vi "String_parsingV3.vi"(4 "input string":string) -> (0 "V3":i32[](array[numeric]), 1 "V2":i32[](array[numeric]), 2 "V1":i32[](array[numeric]))   [LabVIEW 2014]
panel:
  out "size(s)":i32
  out "input test":u8[](array[numeric])
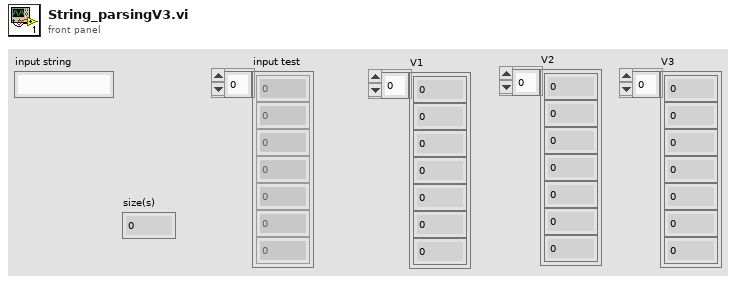
[diagram p1: front panel]
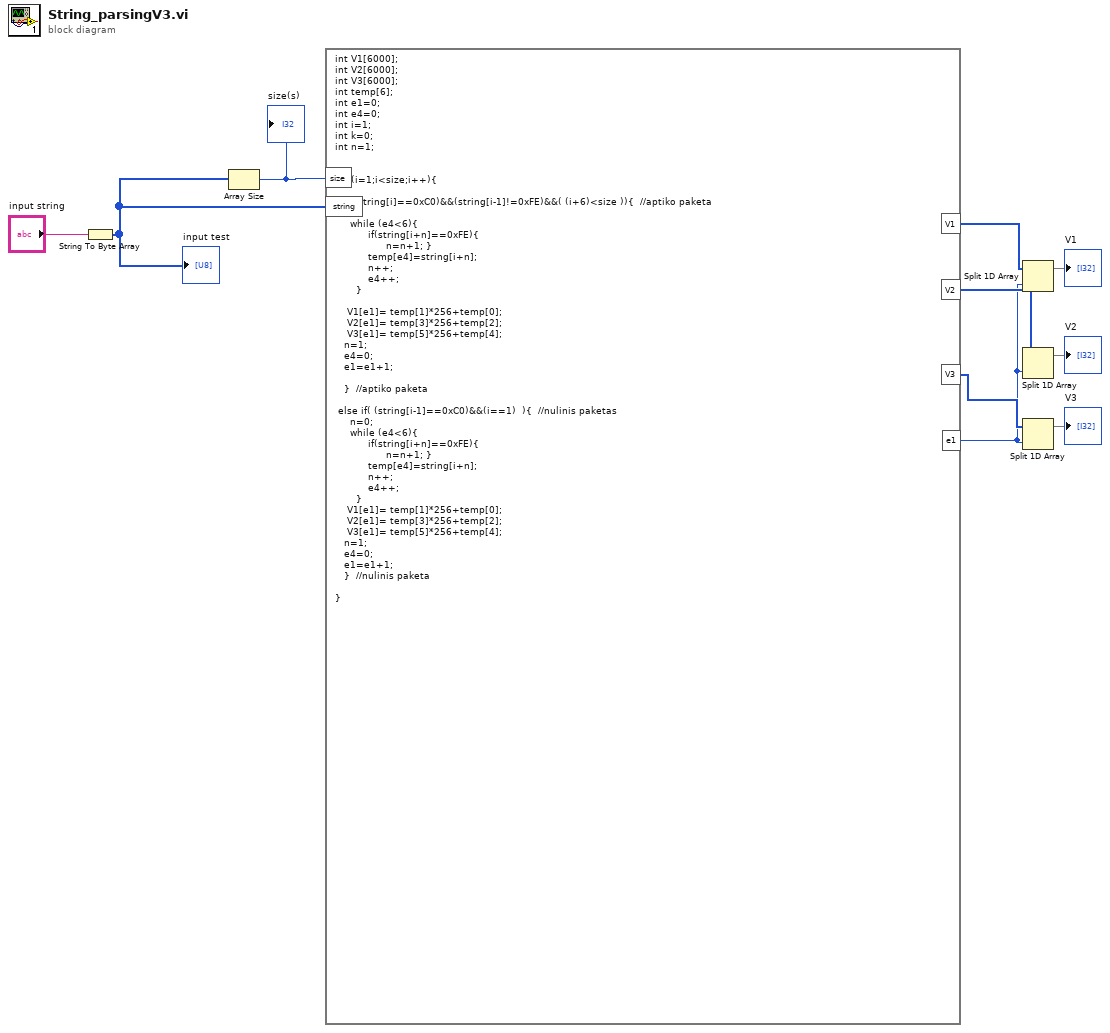
[diagram p0: block diagram]
diagram:
  n1 = String To Byte Array(string="input string") -> (unsigned byte array=w10:u8[])
  "input test" <- w10
  n2 = Array Size(array=w10) -> (size(s)=w9:i32)
  "size(s)" <- w9
  n3 = formula code="int V1[6000];\nint V2[6000];\nint V3[6000];\nint temp[6];\nint e1=0;\nint e4=0;\nint i=1;\nint k=0;\nint n=1;\n\n\nfor (i=1;i<size;i++){\n \n  if( (string[i]==0xC0)&&(string[i-1]!=0xFE)&&( (i+6)<size )){  //aptiko paketa\n\n     while (e4<6){\n           if(string[i+n]==0xFE){\n                 n=n+1; }\n           temp[e4]=string[i+n];\n           n++; \n           e4++;\n       }\n   \n    V1[e1]= temp[1]*256+temp[0];\n    V2[e1]= temp[3]*256+temp[2];\n    V3[e1]= temp[5]*256+temp[4];\n   n=1;\n   e4=0;\n   e1=e1+1;\n   \n   }  //aptiko paketa\n\n else if( (string[i-1]==0xC0)&&(i==1)  ){  //nulinis paketas\n     n=0;\n     while (e4<6){\n           if(string[i+n]==0xFE){\n                 n=n+1; }\n           temp[e4]=string[i+n];\n           n++; \n           e4++;\n       }\n    V1[e1]= temp[1]*256+temp[0];\n    V2[e1]= temp[3]*256+temp[2];\n    V3[e1]= temp[5]*256+temp[4];\n   n=1;\n   e4=0;\n   e1=e1+1;\n   }  //nulinis paketa\n\n}"("string"=w10, "size"=w9) -> ("V1"=w7:i32[], "V2"=w3:i32[], "V3"=w2:i32[], "e1"=w1:i32)
  n4 = Split 1D Array(array=w7, index=w1) -> (first subarray=→"V1":i32[])  [unwired: 1 out]
  n5 = Split 1D Array(array=w3, index=w1) -> (first subarray=→"V2":i32[])  [unwired: 1 out]
  n6 = Split 1D Array(array=w2, index=w1) -> (first subarray=→"V3":i32[])  [unwired: 1 out]
